vi "Menu Init.vi"(8 "error in (no error)":errorcluster, 11 "IDE simple in":refnum<class "LF2R IDE.lvclass">) -> (0 "error out":errorcluster, 3 "IDE simple out":refnum<class "LF2R IDE.lvclass">)   [LabVIEW 2018, in "LF2R IDE.lvlib" / "LF2R IDE.lvclass"]
uses:
  LF2R IDE.lvclass
  LF2R IDE.lvclass/LF2R IDE.ctl
  <userlib>/_MGI/Menu Building/MenuTypes/Vi/VI.vi
  <userlib>/_MGI/Menu Building/MenuTypes/Vi/MGI_VI.lvclass
  <userlib>/_MGI/Menu Building/MenuTypes/MGI_Menu.lvclass
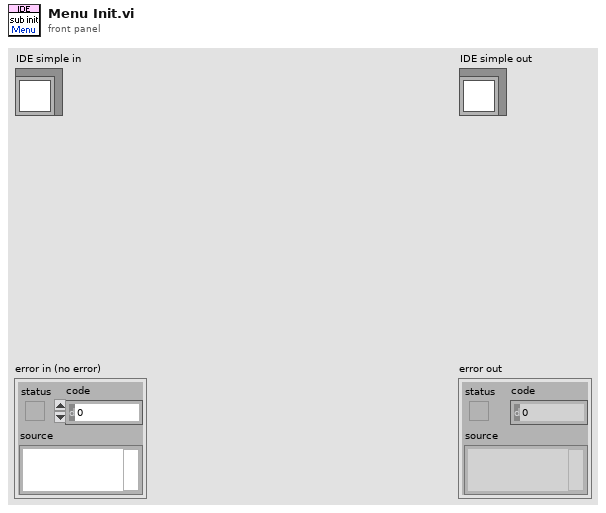
[diagram p1: front panel]
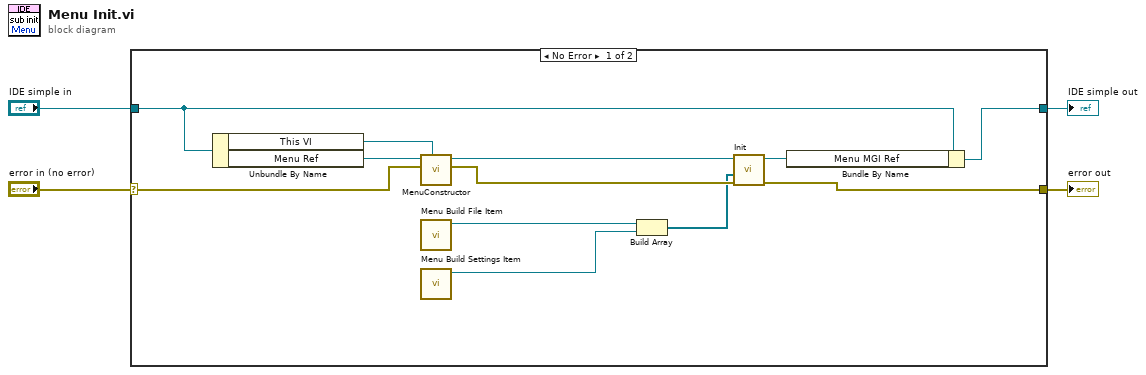
[diagram p0: block diagram]
diagram:
  n1 = case shown="No Error" "error in (no error)" {
    selector: "error in (no error)" -> [w13 w18]
    tunnel: [w8 w18] -> w3
    tunnel: [w11 w17] -> w1
    tunnel: "IDE simple in" -> [w14 w17]
    frame No Error {
      n2 = Unbundle By Name(w14) -> ("This VI"=w15:refnum<vi>, "Menu Ref"=w16:refnum<k9>)
      n3 = call-poly <userlib>:"MenuConstructor.vi"("Menu VI"=w15, "error in (no error)"=w13, "menu reference"=w16) -> ("error out"=w12:errorcluster, "VI"=w10:refnum<class "MGI_VI.lvclass">)  [unwired: 7 in]
      n4 = call "Menu Build File Item.vi"() -> ("Menu File Item"=w7:refnum<data-value>)  [unwired: 11 in]
      n5 = call "Menu Build Settings Item.vi"() -> ("Menu Settings Item"=w5:refnum<data-value>)  [unwired: 11 in]
      n6 = Build Array(w7, w5) -> (w6:refnum<data-value>[])
      n7 = call-dynamic "Init.vi"("error in (no error)"=w12, "Menu Items"=w6, "Menu in"=w10) -> ("error out"=w8:errorcluster, "Menu out"=w9:refnum<class "MGI_VI.lvclass">)  [unwired: 6 in, 1 out]
      n8 = Bundle By Name(cluster=w14, "Menu MGI Ref"=w9) -> (w11:refnum<class "LF2R IDE.lvclass">)
    }
    frame Error {
    }
  }
  "error out" <- w3
  "IDE simple out" <- w1
